vi "EF_GetFeaturesVectorVariance.vi"(8 "error in (no error)":errorcluster, 11 "Array Of Waveforms in":waveform(dbl)[](array[waveform])) -> (0 "error out":errorcluster, 3 "Features Array out":dbl[][](array[numeric]))   [LabVIEW 2016, in "Feature Extraction.lvlib"]
uses:
  Feature Extraction.lvlib
  <vilib>/Analysis/NI_AALBase.lvlib
panel:
  # "This VI is a part of BCI Design library, http://www.ru-bci.org \nCopyright © 2020, Sotnikov Peter, All rights reserved. License: GNU GPLv3"
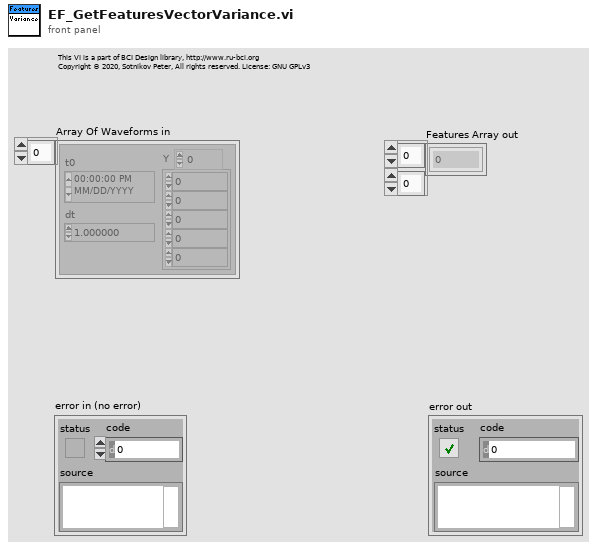
[diagram p1: front panel]
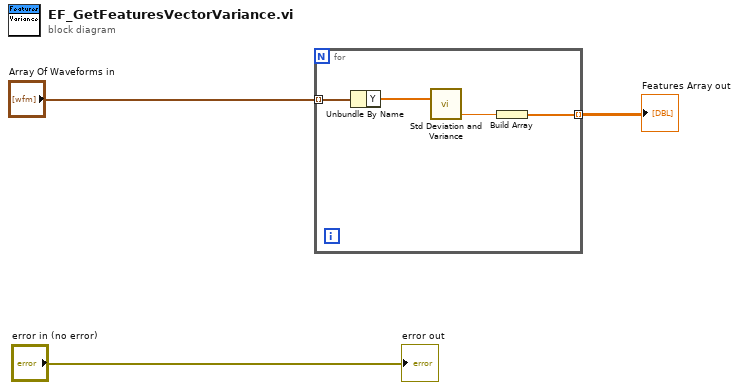
[diagram p0: block diagram]
diagram:
  n1 = for {
    tunnel: "Array Of Waveforms in" -> [w7] mode=indexing
    tunnel: [w4] -> w3 mode=indexing
    n2 = Unbundle By Name(w7) -> ("Y"=w6:dbl[])
    n3 = call <vilib>:"Std Deviation and Variance.vi"("X"=w6) -> ("variance"=w5:dbl)  [unwired: 1 in, 2 out]
    n4 = Build Array(w5) -> (w4:dbl[])
  }
  "Features Array out" <- w3
  "error out" <- "error in (no error)"
